vi "kvCanError.vi"(1 "error code":i32) -> (0 "error out":errorcluster)   [LabVIEW 2022 SP3]
doc: "This VI converts a CAN error code to the \"error out\" cluster object."
uses:
  canlib32.dll
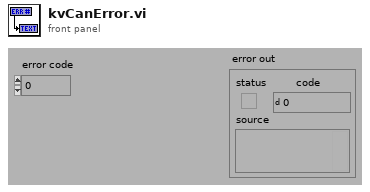
[diagram p1: front panel]
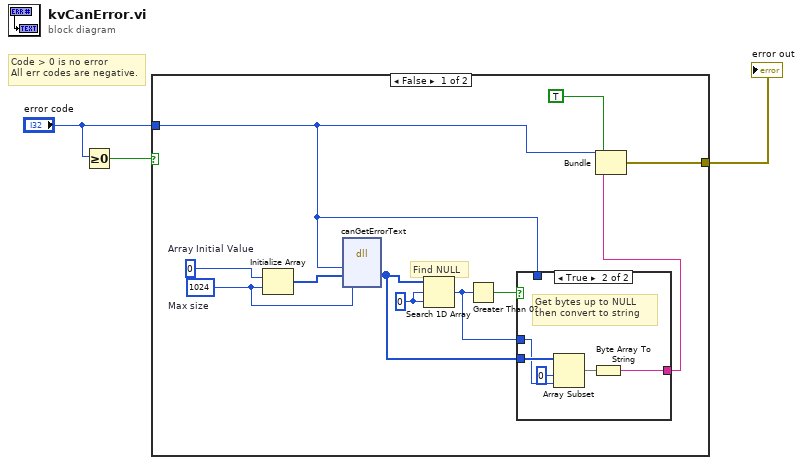
[diagram p0: block diagram]
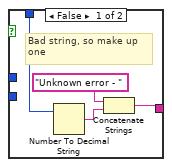
[diagram p2: hidden frame]
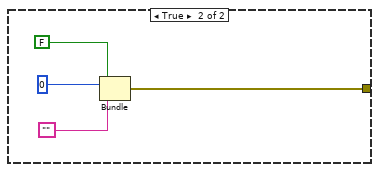
[diagram p3: hidden frame]
diagram:
  # "Code > 0 is no error\nAll err codes are negative."
  n1 = Greater Or Equal To 0?(x="error code") -> (x >= 0?=w3:bool)
  n2 = case shown="False" w3 {
    tunnel: [w13 w24] -> w2
    tunnel: "error code" -> [w5 _]
    frame False {
      w9 = 0
      w10 = 1024  # Max size
      w12 = 0  # Array Initial Value
      # "Find NULL"
      n3 = Initialize Array(w12, w10) -> (w11:i32[])
      n4 = dll-call lib="canlib32.dll" fn="canGetErrorText"("err"=w5, "buf"=w11, "bufsiz"=w10) -> ("buf"=w6:u8[])  [unwired: 6 in, 2 out]
      n5 = Search 1D Array(1D array=w6, element=w9, start index (0)=w9) -> (index of element=w7:i32)
      n6 = Greater Than 0?(x=w7) -> (x > 0?=w8:bool)
      n7 = case shown="True" w8 {
        tunnel: w7 -> [_ w22]
        tunnel: w6 -> [_ w23]
        tunnel: [w15 w19] -> w4
        tunnel: w5 -> [w18 _]
        frame False {
          # "Bad string, so make up\none"
          n8 = Number To Decimal String(number=w18) -> (decimal integer string=w16:string)  [unwired: 1 in]
          n9 = Concatenate Strings("Unknown error - ", w16) -> (w15:string)
        }
        frame True {
          # "Get bytes up to NULL\nthen convert to string"
          n10 = Array Subset(array=w23, index=0, length=w22) -> (w20:u8[])
          n11 = Byte Array To String(unsigned byte array=w20) -> (string=w19:string)
        }
      }
      n12 = Bundle(TRUE, "error code"=w5, "string"=w4) -> (w13:cluster{bool, "error code":i32, "string":string})  [unwired: 1 in]
    }
    frame True {
      n13 = Bundle(FALSE, 0, "") -> (w24:errorcluster)  [unwired: 1 in]
    }
  }
  "error out" <- w2
